vi "HandleAlarms.vi"(0 "Stand in":refnum<class "Stand.lvclass">, 11 "error in (no error)":errorcluster) -> (4 "Stand out":refnum<class "Stand.lvclass">, 13 "dt handle alarms":u32, 15 "error out":errorcluster)   [LabVIEW 2019, in "Stand.lvclass"]
uses:
  Stand.lvclass
  D:/GIT H4000/H4000/src/Device_class/Device.lvclass
  Stand.lvclass/Stand.ctl
  DI_class/DI.lvclass/DI.ctl
  DA_class/DA.lvclass/DA.ctl
  Proccess_class/Proccess.lvclass/Proccess.ctl
  Device_class/Device.lvclass/Device.ctl
  DO_class/DO.lvclass/DO.ctl
  AI_class/AI.lvclass/AI.ctl
  TypeDef/Mode.ctl
  Valve DIR.ctl
  8a3fcd2b-4666-49f3-a38c-8131cd830bc1.vi
  DA_class/UpdateDa.vi
  DI_class/Get_DI.vi
  Device_class/GetFPGA.vi
  AI_class/SetEnable.vi
  DO_class/Read DO.vi
  DoValve.vi
  subvis/bool_change.vi
  DA_class/private/write_to_db.vi
  DoValve.vi/e7d2c9dc-ba67-4685-b926-bcce34aa2778.vi
  DoValve.vi/628819af-fd07-4303-9780-3ddd467101db.vi
  Proccess_class/GetNames.vi
  Proccess_class/GetLogger.vi
  DA_class/DA.lvclass
  D:/GIT H4000/H4000/src/Proccess_class/Proccess.lvclass
  Logger_class/WriteEvent.vi
  Const All Valve.vi
  FPGA_API_class/FPGA API.lvclass
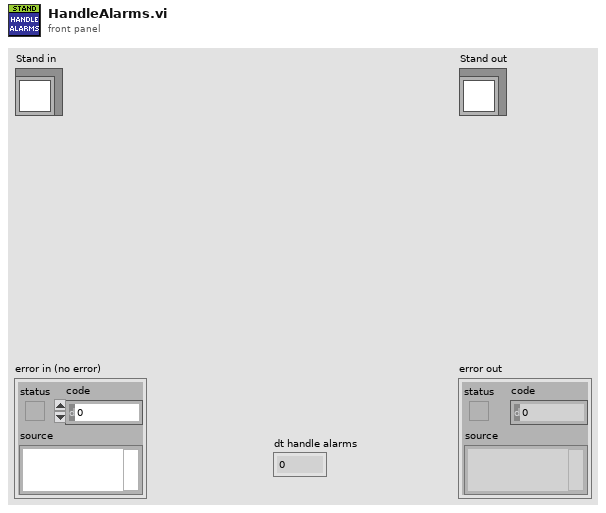
[diagram p1: front panel]
types:
  T1 = typedef "Valve DIR.ctl" = enum16{"Air Valves: Open (DUT Filling)", "Air Valves: Open (Chamber Filling)", "Air Valves: Open (Pump Pressure DUT)", "Air Valves: Open (Pump Pressure Chamber)", "Air Valves: Open (Haskel Pressure DUT)", "Air Valves: Open (Haskel Pressure Chamber)", "Air Valves: Open (Slow Release DUT)", "Air Valves: Open (Slow Release Chamber)", "Air Valves: Open (Fast Release DUT)", "Air Valves: Open (Fast Release Chamber)", "Air Valves: Open (Emergency Release DUT and Chamber)", "Air Valves: Leak Hi (Chamber)", "Air Valves: Leak Hi (DUT)", "Air Valves: Backpressure (Chamber)", "Air Valves: Backpressure (DUT)", "Air Valves: Fully Closed", "Air Valves: Open 33.7"}
  T2 = typedef "Mode.ctl" = enum16{"IDLE", "FILLING", "EXECUTE_SP", "DRAIN"}
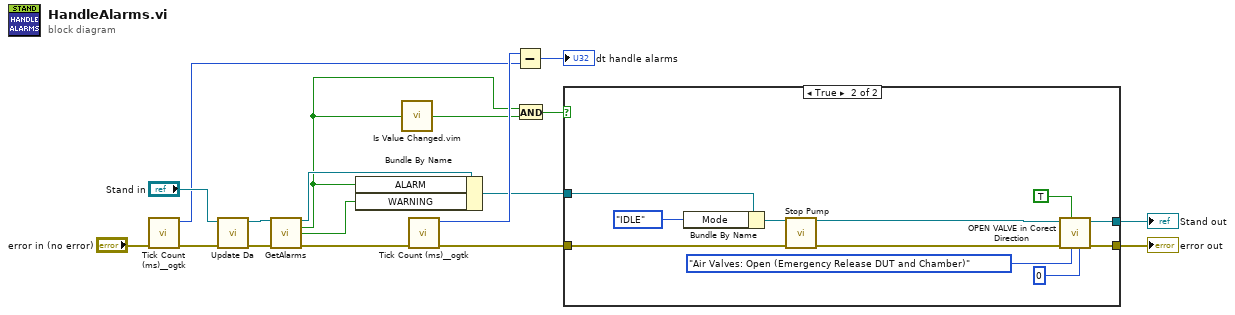
[diagram p0: block diagram]
diagram:
  n1 = call <userlib>:"Tick Count (ms)__ogtk.vi"("error in (no error)"="error in (no error)") -> ("error out"=w12:errorcluster, "millisecond timer value"=w10:u32)  [unwired: 9 in]
  n2 = call "Update Da.vi"("error in (no error)"=w12, "Stand in"="Stand in") -> ("error out"=w15:errorcluster, "Stand out"=w16:refnum<class "Stand.lvclass">)  [unwired: 8 in]
  n3 = call-dynamic "GetAlarms.vi"("reference in"=w16, "error in (no error)"=w15) -> ("reference out"=w14:refnum<class "Stand.lvclass">, "Alarm"=w2:bool, "Warning"=w1:bool, "error out"=w8:errorcluster)  [unwired: 10 in]
  n4 = Bundle By Name(cluster=w14, "ALARM"=w2, "WARNING"=w1) -> (w3:refnum<class "Stand.lvclass">)
  n5 = call "Is Value Changed.vim"("value"=w2) -> ("changed or first call?"=w6:bool)
  n6 = call <userlib>:"Tick Count (ms)__ogtk.vi"("error in (no error)"=w8) -> ("error out"=w5:errorcluster, "millisecond timer value"=w11:u32)  [unwired: 9 in]
  n7 = Subtract(x=w11, y=w10) -> (x-y=→"dt handle alarms":u32)
  n8 = And(x=w2, y=w6) -> (x .and. y?=w7:bool)
  n9 = case shown="True" w7 {
    tunnel: w3 -> [w20 w30]
    tunnel: [w20 w25] -> w18
    tunnel: w5 -> [w19 w28]
    tunnel: [w19 w24] -> w4
    frame False {
    }
    frame True {
      n10 = Bundle By Name(cluster=w30, "Mode"=Mode."IDLE" ("Data.Mode")) -> (w29:refnum<class "Stand.lvclass">)
      n11 = call "Stop Pump.vi"("reference in"=w29, "error in (no error)"=w28) -> ("reference out"=w27:refnum<class "Stand.lvclass">, "error out"=w26:errorcluster)  [unwired: 11 in, 1 out]
      n12 = call "OPEN VALVE in Corect Direction.vi"("time after close"=u32 0, "Valve DIR"=Valve_DIR."Air Valves: Open (Emergency Release DUT and Chamber)", "changed or first call?"=TRUE, "error in (no error)"=w26, "Stand in"=w27) -> ("error out"=w24:errorcluster, "Stand out"=w25:refnum<class "Stand.lvclass">)  [unwired: 4 in, 1 out]
    }
  }
  "error out" <- w4
  "Stand out" <- w18
